vi "CreateCouplingCapFile.vi"(0 "Filename IN":string, 1 "Pass rate":dbl format="%.2f", 2 "No of strips":i32, 3 "cap array in":dbl[](array[numeric]) format="%.2f", 4 "Segment:":i32, 5 "Defect Flag Array":i32[][](array[numeric])) -> (6 "DBFileName OUT":string, 7 "passed":bool, 8 "DBfileSaved?":bool)   [LabVIEW 2013]
uses:
  global/newtest.vi
panel:
  in  "Anneal Time:":dbl
  in  "Radiation Dose:":dbl
  out "Deviation [pF]":dbl
  out "Mean Capacitance [pF]":dbl
  in  "Add comment":bool
  in  "cancel":bool
  in  "create file":bool
  out "% good strips:":dbl format="%.2f"
  out "Run Number:":string
  out "Date:":string
  out "Location:":string
  out "Operator:":string
  out "Passed?":bool
  out "SCT Serial No.:":string
  out "Comments?":string
  in  "Problem?":bool
  # "Write Coupling Capacitor DataBase File"
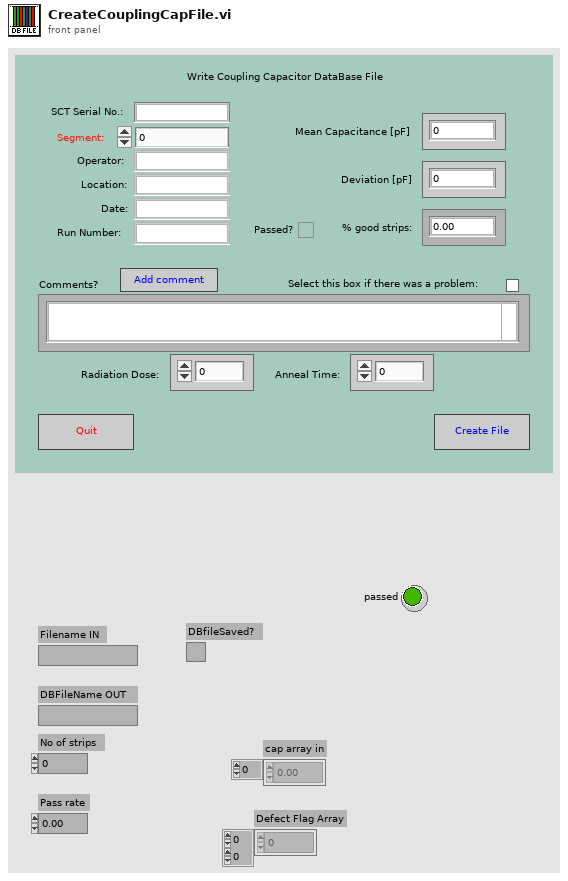
[diagram p1: front panel]
types:
  T1 = cluster{"Serial Number":string, "Operator":string, "Run number":string, "Date":string, "lookup":u16, "Device type":string}
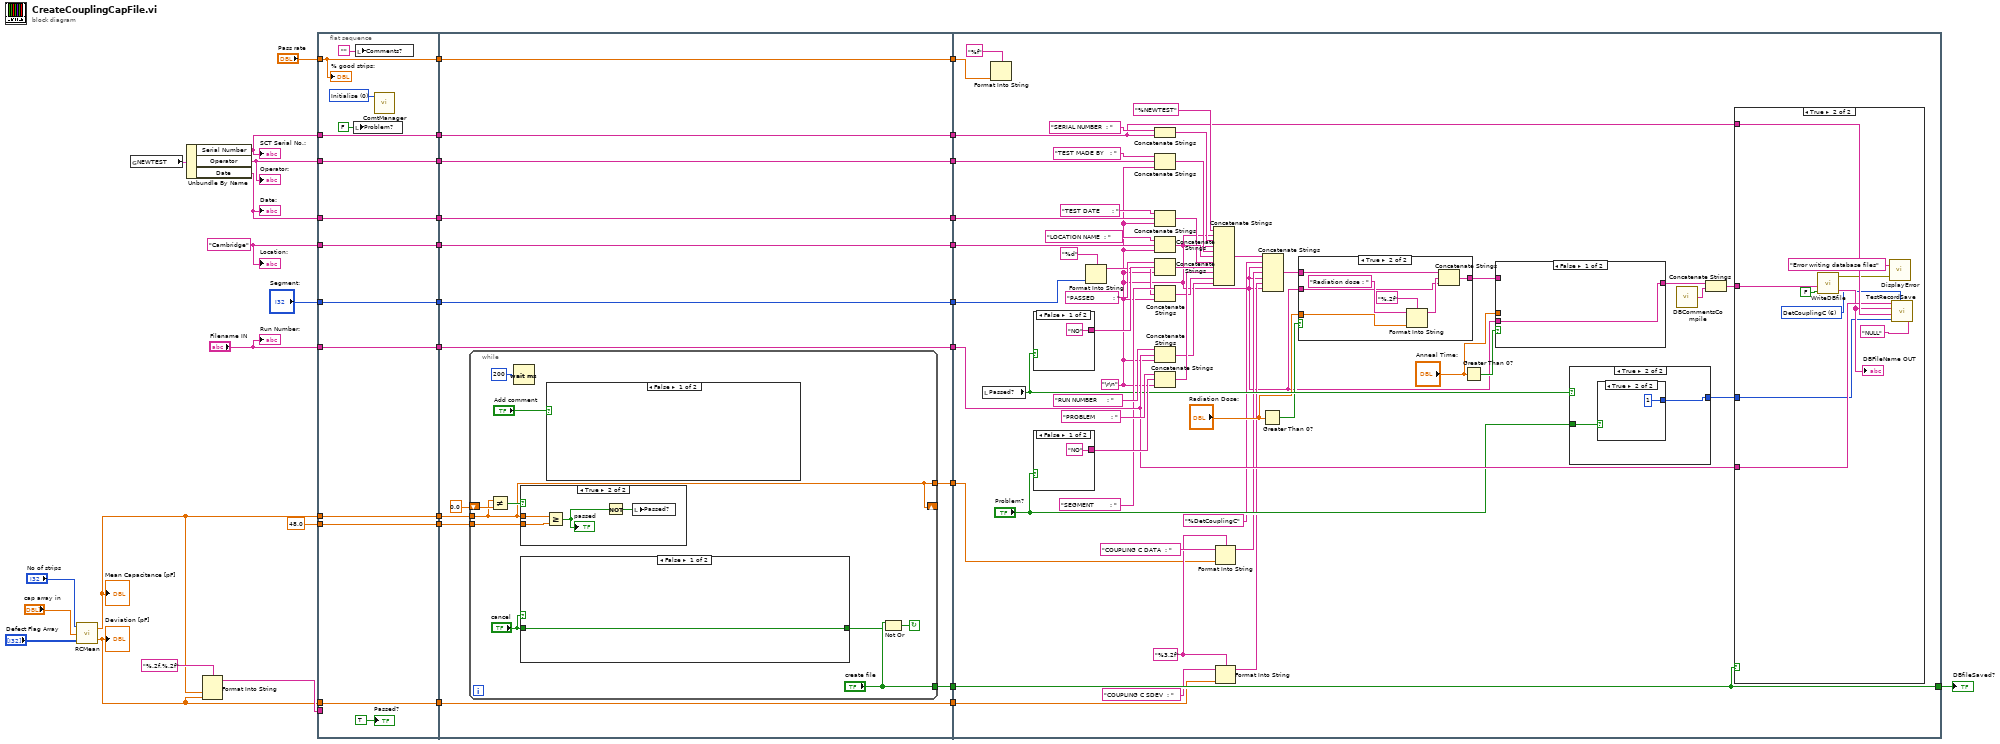
[diagram p0: block diagram]
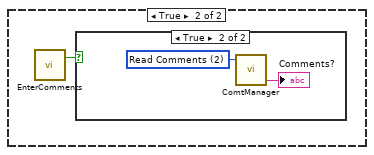
[diagram p3: hidden frame]
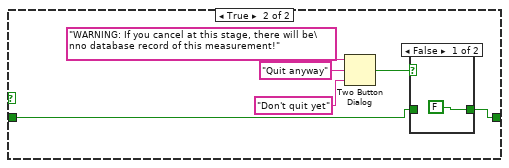
[diagram p5: hidden frame]
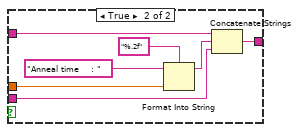
[diagram p7: hidden frame]
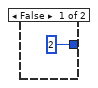
[diagram p9: hidden frame]
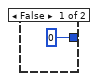
[diagram p10: hidden frame]
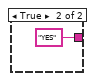
[diagram p12: hidden frame]
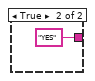
[diagram p13: hidden frame]
diagram:
  w33 = "Cambridge" ("Location:")
  n1 = call "RCMean.vi"("Defect Flag array IN"="Defect Flag Array", "data array in"="cap array in", "No of strips"="No of strips") -> ("standard deviation"=w21:dbl, "mean"=w23:dbl)
  "Mean Capacitance [pF]" <- w23
  "Deviation [pF]" <- w21
  n2 = global read "newtest.vi" "NEWTEST"() -> (w37:T1)
  n3 = Unbundle By Name(w37) -> ("Serial Number"=w36:string, "Operator"=w35:string, "Date"=w34:string)
  "SCT Serial No.:" <- w36
  "Operator:" <- w35
  "Date:" <- w34
  n4 = Format Into String(format string="%.2f,%.2f" ("Format String"), w23, w21) -> (resulting string=w24:string)  [unwired: 2 in, 1 out]
  n5 = flat-sequence {
    tunnel: w36 -> [w46]
    tunnel: [w46] -> w20
    tunnel: w35 -> [w45]
    tunnel: [w45] -> w19
    tunnel: w34 -> [w44]
    tunnel: [w44] -> w18
    tunnel: w33 -> [w43]
    tunnel: [w43] -> w17
    tunnel: "Filename IN" -> [w42]
    tunnel: [w42] -> w16
    tunnel: "Pass rate" -> [w49]
    tunnel: [w49] -> w15
    tunnel: "Segment:" -> [w41]
    tunnel: [w41] -> w14
    tunnel: w24 -> [_]
    tunnel: w23 -> [w40]
    tunnel: [w40] -> w13
    tunnel: 48.0 -> [w39]
    tunnel: [w39] -> w12
    tunnel: w21 -> [w38]
    tunnel: [w38] -> w11
    tunnel: w20 -> [w59]
    tunnel: [w59] -> w10
    tunnel: w19 -> [w58]
    tunnel: [w58] -> w9
    tunnel: w18 -> [w57]
    tunnel: [w57] -> w8
    tunnel: w17 -> [w56]
    tunnel: [w56] -> w7
    tunnel: w16 -> [w55]
    tunnel: [w55] -> w6
    tunnel: w15 -> [w54]
    tunnel: [w54] -> w5
    tunnel: w14 -> [w53]
    tunnel: [w53] -> w4
    tunnel: w13 -> [w63]
    tunnel: w12 -> [w62]
    tunnel: [w61] -> w3
    tunnel: w11 -> [w52]
    tunnel: [w52] -> w2
    tunnel: [w64] -> w1
    tunnel: w10 -> [w119]
    tunnel: w9 -> [w131]
    tunnel: w8 -> [w130]
    tunnel: w7 -> [w129]
    tunnel: [w125] -> w32
    tunnel: w6 -> [w118]
    tunnel: w5 -> [w122]
    tunnel: w4 -> [w113]
    tunnel: w3 -> [w92]
    tunnel: w2 -> [w100]
    tunnel: w1 -> [w125]
    frame #0 {
      w48 = u16 0 items=["Initialise", "Add comment", "Read Comments"] ("Action")
      n6 = local write "Problem?"(FALSE ("Problem?")) -> ()
      n7 = local write "Comments?"("") -> ()
      n8 = call "ComtManager.vi"("Action"=w48) -> ()  [unwired: 2 in, 3 out]
      "Passed?" <- TRUE
      "% good strips:" <- w49
    }
    frame #1 {
      n9 = while {
        tunnel: ["create file"] -> w64
        tunnel: w63 -> [w65]
        tunnel: w62 -> [w68]
        shift-right: [w65] -> _
        shift-left: 0.0 -> [w67]
        tunnel: [w65] -> w61
        stop <- w74 continue-if-true
        n10 = Not Equal?(x=w65, y=w67) -> (x != y?=w66:bool)
        n11 = Wait (ms)(milliseconds to wait=u32 200) -> ()  [unwired: 1 out]
        n12 = case shown="True" w66 {
          tunnel: w68 -> [_ w78]
          tunnel: w65 -> [_ w77]
          frame False {
          }
          frame True {
            n13 = Greater Or Equal?(x=w77, y=w78) -> (x >= y?=w75:bool)
            "passed" <- w75
            n14 = Not(x=w75) -> (.not. x?=w76:bool)
            n15 = local write "Passed?"(w76) -> ()
          }
        }
        n16 = case shown="False" "cancel" {
          tunnel: [w82 w84] -> w72
          tunnel: "cancel" -> [w82 w83]
          frame False {
          }
          frame True {
            n17 = Two Button Dialog(message="WARNING: If you cancel at this stage, there will be\nno database record of this measurement!", 1:"Don't quit yet" ("F button name (\"Cancel\")"), 2:"Quit anyway" ("T button name (\"OK\")")) -> (T button?=w85:bool)
            n18 = case shown="False" w85 {
              tunnel: [FALSE w90] -> w84
              tunnel: w83 -> [_ w90]
              frame False {
              }
              frame True {
              }
            }
          }
        }
        n19 = case shown="False" "Add comment" {
          frame False {
          }
          frame True {
            n20 = call "EnterComments.vi"() -> ("update?"=w79:bool)  [unwired: 4 in]
            n21 = case shown="True" w79 {
              frame False {
              }
              frame True {
                w81 = u16 2 items=["Initialise", "Add comment", "Read Comments"] ("Action")
                n22 = call "ComtManager.vi"("Action"=w81) -> ("Comment out"=→"Comments?":string)  [unwired: 2 in, 2 out]
              }
            }
          }
        }
        n23 = Not Or(1:w72, 2:"create file") -> (0:w74:bool)
      }
    }
    frame #2 {
      w103 = "%3.2f"
      w96 = "\r\n"
      n24 = local read "Passed?"() -> (w110:bool)
      n25 = Format Into String(format string="%f", w122) -> ()  [unwired: 2 in, 2 out]
      n26 = case shown="False" w110 {
        tunnel: ["NO" "YES"] -> w128
        frame False {
        }
        frame True {
        }
      }
      n27 = case shown="False" "Problem?" {
        tunnel: ["NO" "YES"] -> w127
        frame False {
        }
        frame True {
        }
      }
      n28 = Format Into String(format string="%d", w113) -> (resulting string=w112:string)  [unwired: 2 in, 1 out]
      n29 = Concatenate Strings("SERIAL NUMBER  : ", w119) -> (w121:string)
      n30 = Concatenate Strings("TEST MADE BY   : ", w131, w96) -> (w136:string)
      n31 = Concatenate Strings("TEST DATE      : ", w130, w96) -> (w134:string)
      n32 = Concatenate Strings("LOCATION NAME  : ", w129, w96) -> (w135:string)
      n33 = Concatenate Strings("PASSED         : ", w128, w96) -> (w133:string)
      n34 = Concatenate Strings("SEGMENT        : " ("string"), w112, w96) -> (w111:string)
      n35 = Concatenate Strings("RUN NUMBER     : ", w118, w96) -> (w123:string)
      n36 = Concatenate Strings("PROBLEM        : ", w127, w96) -> (w132:string)
      n37 = Concatenate Strings("%NEWTEST", w96, w121, w96, w136, w135, w134, w133, w132, w111, w123) -> (w107:string)
      n38 = Format Into String(format string=w103, initial string="COUPLING C DATA  : ", w92) -> (resulting string=w102:string)  [unwired: 1 in, 1 out]
      n39 = Format Into String(format string=w103, initial string="COUPLING C SDEV  : ", w100) -> (resulting string=w101:string)  [unwired: 1 in, 1 out]
      n40 = Greater Than 0?(x="Radiation Dose:") -> (x > 0?=w109:bool)
      n41 = Concatenate Strings(w107, "%DetCouplingC", w96, w102, w96, w101, w96) -> (w91:string)
      n42 = case shown="True" w109 {
        tunnel: "Radiation Dose:" -> [_ w157]
        tunnel: [w151 w154] -> w99
        tunnel: w96 -> [w151 w153]
        tunnel: w91 -> [_ w152]
        frame False {
        }
        frame True {
          n43 = Format Into String(format string="%.2f", initial string="Radiation dose : ", w157) -> (resulting string=w155:string)  [unwired: 1 in, 1 out]
          n44 = Concatenate Strings(w152, w155, w153) -> (w154:string)
        }
      }
      n45 = Greater Than 0?(x="Anneal Time:") -> (x > 0?=w98:bool)
      n46 = case shown="False" w98 {
        tunnel: "Anneal Time:" -> [_ w149]
        tunnel: w96 -> [w143 w147]
        tunnel: [w143 w145] -> w95
        tunnel: w99 -> [_ w144]
        frame False {
        }
        frame True {
          n47 = Format Into String(format string="%.2f", initial string="Anneal time    : ", w149) -> (resulting string=w146:string)  [unwired: 1 in, 1 out]
          n48 = Concatenate Strings(w144, w146, w147) -> (w145:string)
        }
      }
      n49 = case shown="True" w110 {
        tunnel: [u16 2 w160] -> w117
        tunnel: "Problem?" -> [_ w161]
        frame False {
        }
        frame True {
          n50 = case shown="True" w161 {
            tunnel: [u16 0 u16 1] -> w160
            frame False {
            }
            frame True {
            }
          }
        }
      }
      n51 = call "DBCommentsCompile.vi"() -> ("Comments out"=w94:string)
      n52 = Concatenate Strings(w95, w94) -> (w93:string)
      n53 = case shown="True" w125 {
        tunnel: w119 -> [_ w172]
        tunnel: w118 -> [_ w171]
        tunnel: w117 -> [_ w169]
        tunnel: w93 -> [_ w164]
        frame False {
        }
        frame True {
          w168 = u16 6 items=["DetIVscan", "DetDefect", "DetVDep", "DetILeak", "VisInspec", "DetInterC", "DetCouplingC", "DetBiasR", "DetAluStripR"] ("File Type")
          n54 = call "WriteDBfile.vi"("String IN"=w164, "UploadRawData?"=FALSE) -> ("error out"=w166:errorcluster, "DBFileName OUT"=w170:string)  [unwired: 4 in, 1 out]
          "DBFileName OUT" <- w170
          n55 = call "DisplayError.vi"("Error In"=w166, "Error String In"="Error writing database files" ("Error String IN")) -> ()
          n56 = call "TestRecordSave.vi"("Local Record"=w171, "Database file reference"=w170, "Serial No."=w172, "Pass flag"=w169, "File Type"=w168, "INFO field"="NULL") -> ()  [unwired: 1 in]
        }
      }
    }
  }
  "Run Number:" <- "Filename IN"
  "Location:" <- w33
  "DBfileSaved?" <- w32
